vi "DataXML init.vi"(8 "error in (no error)":errorcluster, 9 "file path":path, 10 "root node name":string="Information", 11 "DataXML in":refnum<class "DataXML.lvclass">) -> (0 "error out":errorcluster, 3 "DataXML out":refnum<class "DataXML.lvclass">)   [LabVIEW 2018, in "DataXML.lvclass"]
uses:
  DataXML.lvclass
  DataXML.lvclass/DataXML.ctl
  <vilib>/xml/Load XML File.vi
  <resource>/objmgr/DOMUserDefRef.rc
  <vilib>/xml/NI_XML.lvlib
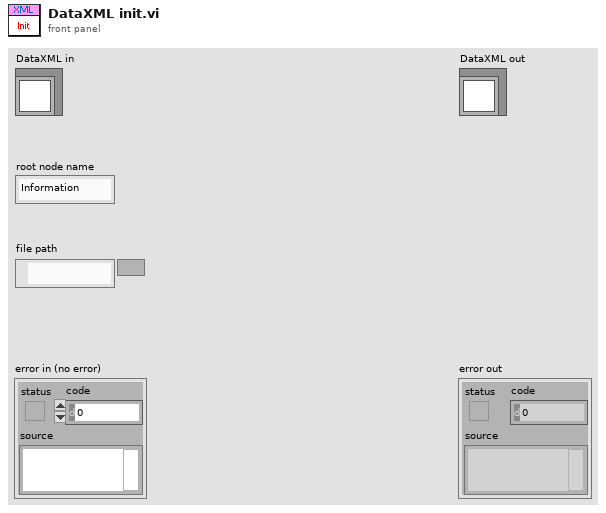
[diagram p1: front panel]
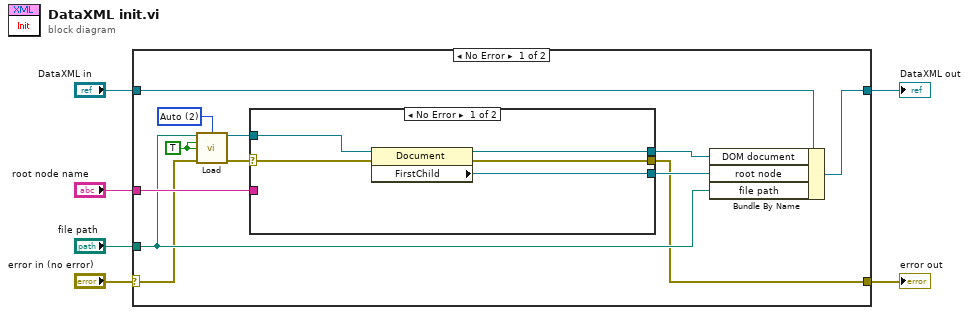
[diagram p0: block diagram]
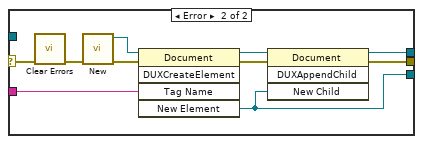
[diagram p2: hidden frame]
diagram:
  n1 = case shown="No Error" "error in (no error)" {
    selector: "error in (no error)" -> [w8 w34]
    tunnel: [w7 w34] -> w5
    tunnel: [w12 w35] -> w3
    tunnel: "DataXML in" -> [w13 w35]
    tunnel: "root node name" -> [w18 _]
    tunnel: "file path" -> [w9 _]
    frame No Error {
      w17 = 2 items=["Never", "Always", "Auto"] ("validate on load (Auto)")
      w16 = TRUE ("process namespaces (False)")
      n2 = call-poly <vilib>:"Load.vi"("path to XML document"=w9, "validate on load (Auto)"=w17, "process namespaces (False)"=w16, "process schema (False)"=w16, "error in (no error)"=w8) -> ("DOM document out"=w14:refnum<k20>, "error out"=w15:errorcluster)  [unwired: 8 in, 1 out]
      n3 = case shown="No Error" w15 {
        selector: w15 -> [w23 w27]
        tunnel: w18 -> [_ w29]
        tunnel: w14 -> [w22 _]
        tunnel: [w21 w26] -> w10
        tunnel: [w20 w25] -> w11
        tunnel: [w19 w24] -> w7
        frame No Error {
          n4 = property class="Document"(reference=w22, error in=w23) -> (reference out=w20:refnum<k20>, error out=w19:errorcluster, "FirstChild"=w21:refnum<k20>)
        }
        frame Error {
          n5 = call <vilib>:"Clear Errors.vi"("error in (no error)"=w27) -> ("error out"=w28:errorcluster)  [unwired: 5 in, 1 out]
          n6 = call <vilib>:"New.vi"("error in (no error)"=w28) -> ("error out"=w32:errorcluster, "DOM document out"=w30:refnum<k20>)  [unwired: 7 out]
          n7 = invoke class="Document" method="DUXCreateElement"(reference=w30, error in=w32, "Tag Name"=w29) -> (reference out=w33:refnum<k20>, error out=w31:errorcluster, "New Element"=w26:refnum<k20>)  [unwired: 2 in, 2 out]
          n8 = invoke class="Document" method="DUXAppendChild"(reference=w33, error in=w31, "New Child"=w26) -> (reference out=w25:refnum<k20>, error out=w24:errorcluster)  [unwired: 1 in, 2 out]
        }
      }
      n9 = Bundle By Name(cluster=w13, "DOM document"=w11, "root node"=w10, "file path"=w9) -> (w12:refnum<class "DataXML.lvclass">)
    }
    frame Error {
    }
  }
  "error out" <- w5
  "DataXML out" <- w3
